vi "PH_Strings.clean array from doubles.vi"(0 "Array Input":string[](array[string])) -> (1 "Array Output":string[](array[string]), 2 "Cleaned Array Output":string[](array[string]))   [LabVIEW 2014, in "PH_Common.lvlib"]
doc: "This VI removes double entries from \"Array Input\". \"Cleaned Array Output\" is additionally freed from empty entries or \"N/A\"s."
uses:
  PH_Common.lvlib
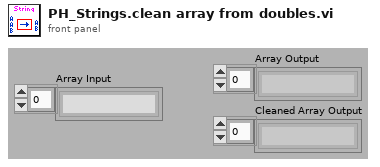
[diagram p1: front panel]
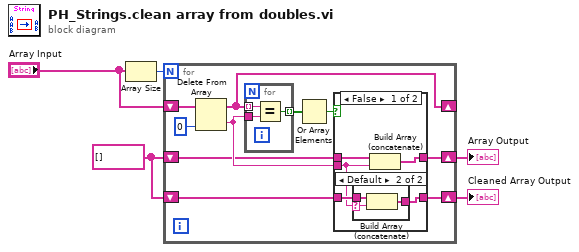
[diagram p0: block diagram]
diagram:
  w1 = string[] [] ("Empty Input")
  n1 = Array Size(array="Array Input") -> (size(s)=w5:i32)
  n2 = for {
    N: w5 -> [_]
    shift-right: [w10] -> w3
    shift-left: w1 -> [w9]
    shift-right: [w8] -> _
    shift-left: "Array Input" -> [w14]
    shift-right: [w7] -> w2
    shift-left: w1 -> [w6]
    n3 = Delete From Array(array=w14, index=0) -> (deleted portion=w11:string, array with subset deleted=w8:string[])  [unwired: 1 in]
    n4 = for {
      tunnel: w11 -> [w28]
      tunnel: w8 -> [w29] mode=indexing
      tunnel: [w27] -> w15 mode=indexing
      n5 = Equal?(x=w29, y=w28) -> (x = y?=w27:bool)
    }
    n6 = Or Array Elements(Boolean array=w15) -> (logical OR=w12:bool)
    n7 = case shown="False" w12 {
      tunnel: w11 -> [w16 _]
      tunnel: [w20 w26] -> w10
      tunnel: w9 -> [w19 w26]
      tunnel: [w18 w25] -> w7
      tunnel: w6 -> [w17 w25]
      frame False {
        n8 = case shown="Default" w16 {
          selector: w16 -> [_ w22]
          tunnel: [w21 w24] -> w18
          tunnel: w17 -> [w21 w23]
          frame "", "N/A" {
          }
          frame Default {
            n9 = Build Array (concatenate)(w23, w22) -> (w24:string[])
          }
        }
        n10 = Build Array (concatenate)(w19, w16) -> (w20:string[])
      }
      frame True {
      }
    }
  }
  "Array Output" <- w3
  "Cleaned Array Output" <- w2
